vi "Get Input Muted.vi"(8 "error in (no error)":errorcluster, 10 "Input Name":string, 11 "OBS in":refnum<class "OBS.lvclass">) -> (0 "error out":errorcluster, 2 "Muted":bool, 3 "OBS out":refnum<class "OBS.lvclass">)   [LabVIEW 2022 SP3, in "obs-websocket-lv.lvlib" / "OBS.lvclass"]
uses:
  OBS.lvclass
  OBS.lvclass/OBS.ctl
  GetInputMute/GetInputMute.lvclass
  RGetInputMute/RGetInputMute.lvclass
  C:/dev/illuminatedg/obs-websocket-lv/obs-websocket-lv/Response/Response.lvclass
  C:/dev/illuminatedg/obs-websocket-lv/obs-websocket-lv/Server Message/Server Message.lvclass
  C:/dev/illuminatedg/obs-websocket-lv/obs-websocket-lv/Message/Message.lvclass
  C:/dev/illuminatedg/obs-websocket-lv/obs-websocket-lv/RGetInputMute/RGetInputMute.lvclass
  C:/dev/illuminatedg/obs-websocket-lv/obs-websocket-lv/Request/Request.lvclass
  C:/dev/illuminatedg/obs-websocket-lv/obs-websocket-lv/Client Message/Client Message.lvclass
  C:/dev/illuminatedg/obs-websocket-lv/obs-websocket-lv/GetInputMute/GetInputMute.lvclass
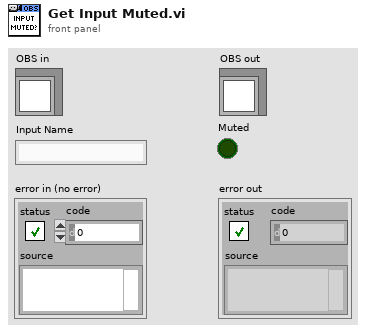
[diagram p1: front panel]
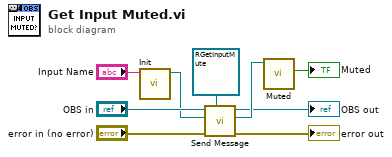
[diagram p0: block diagram]
diagram:
  n1 = call "Init.vi"("Input Name"="Input Name") -> ("GetInputMute out"=w6:refnum<class "GetInputMute.lvclass">)  [unwired: 9 in, 1 out]
  n2 = call "Send Message.vi"("Response Type (None)"=refnum<class "RGetInputMute.lvclass"> refnum ("obs-websocket-lv.lvlib:RGetInputMute.lvclass"), "error in (no error)"="error in (no error)", "Client Message"=w6, "OBS in"="OBS in") -> ("error out"=→"error out":errorcluster, "Response"=w4:refnum<class "RGetInputMute.lvclass">, "OBS out"=→"OBS out":refnum<class "OBS.lvclass">)  [unwired: 4 in, 1 out]
  n3 = call "Muted.vi"("RGetInputMute in"=w4) -> ("Muted"=→"Muted":bool)  [unwired: 8 in, 2 out]
